vi "Actor Core.vi"(8 "error in":errorcluster, 11 "Electronic Load in":refnum<class "Electronic Load.lvclass">) -> (0 "error out":errorcluster, 3 "Actor out":refnum<class "Actor.lvclass">)   [LabVIEW 2019, in "Electronic Load.lvlib" / "Electronic Load.lvclass"]
doc: "The instrument actor core is only here to distribute panel resolution settings to children classes."
uses:
  Library/Electronic Load.lvclass
  C:/Users/Public/Documents/Development/builds/Instruments/Instruments.lvlibp/Library/Instruments.lvclass
  builds/Engine/Actor Framework.lvlibp/1abvi3w/vi.lib/ActorFramework/Actor/Actor.lvclass
  Custom Controls/E-Load Function.ctl
  Custom Controls/E-Load Mode.ctl
  Custom Controls/Trigger Settings.ctl
  Custom Controls/OCP Settings.ctl
  Custom Controls/Status_Flags.ctl
  Library/Electronic Load.lvclass/Electronic Load.ctl
  Electronic Load Messages/Write Output Enable Msg/Write Output Enable Msg.lvclass/Write Output Enable Msg.ctl
  Electronic Load Messages/Write Input Level Msg/Write Input Level Msg.lvclass/Write Input Level Msg.ctl
  Electronic Load Messages/Write Mode Msg/Write Mode Msg.lvclass/Write Mode Msg.ctl
  Electronic Load Messages/Write Slew Rate Msg/Write Slew Rate Msg.lvclass/Write Slew Rate Msg.ctl
  Electronic Load Messages/Write Pulse Enable Msg/Write Pulse Enable Msg.lvclass/Write Pulse Enable Msg.ctl
  Electronic Load Messages/Write Pulse Mode Msg/Write Pulse Mode Msg.lvclass/Write Pulse Mode Msg.ctl
  Electronic Load Messages/Write Pulse Initial Msg/Write Pulse Initial Msg.lvclass/Write Pulse Initial Msg.ctl
  Electronic Load Messages/Write Transient Msg/Write Transient Msg.lvclass/Write Transient Msg.ctl
  Electronic Load Messages/Write Pulse Sample Interval Msg/Write Pulse Sample Interval Msg.lvclass/Write Pulse Sample Interval Msg.ctl
  Electronic Load Messages/Write Pulse Width Msg/Write Pulse Width Msg.lvclass/Write Pulse Width Msg.ctl
  Electronic Load Messages/Write Pulse Delay Msg/Write Pulse Delay Msg.lvclass/Write Pulse Delay Msg.ctl
  Electronic Load Messages/Write Pulse Data Points Msg/Write Pulse Data Points Msg.lvclass/Write Pulse Data Points Msg.ctl
  Electronic Load Messages/Write Pulse Slew Msg/Write Pulse Slew Msg.lvclass/Write Pulse Slew Msg.ctl
  Electronic Load Messages/Write OCP Enable Msg/Write OCP Enable Msg.lvclass/Write OCP Enable Msg.ctl
  Electronic Load Messages/Write OCP Level Msg/Write OCP Level Msg.lvclass/Write OCP Level Msg.ctl
  Electronic Load Messages/Write OCP Delay Msg/Write OCP Delay Msg.lvclass/Write OCP Delay Msg.ctl
  Electronic Load Messages/Write Active Channel Msg/Write Active Channel Msg.lvclass/Write Active Channel Msg.ctl
  Private/GUI/Write Channels_Ref.vi
  Private/GUI/Write Settings_Ref.vi
  Private/GUI/Write Trigger_Ref.vi
  Private/GUI/Write Measured_Table.vi
  Private/GUI/Write OCP_Settings_Ref.vi
  Private/GUI/Write Trigger_TargetsRef.vi
  Private/GUI/Write Status_Flags_Ref.vi
  builds/Instruments/Instruments.lvlibp/Accessors/Write Snapshot Refnum.vi
  builds/Instruments/Instruments.lvlibp/Accessors/Write Graph_Ref.vi
  builds/Engine/Actor Framework.lvlibp/1abvi3w/vi.lib/ActorFramework/Message Enqueuer/Enqueue.vi
  Electronic Load Messages/Write Output Enable Msg/Write Output Enable Msg.lvclass
  Electronic Load Messages/Write Input Level Msg/Write Input Level Msg.lvclass
  Electronic Load Messages/Write Mode Msg/Write Mode Msg.lvclass
  Electronic Load Messages/Write Slew Rate Msg/Write Slew Rate Msg.lvclass
  Electronic Load Messages/Reset Eload Msg/Reset Eload Msg.lvclass
  Electronic Load Messages/Write Pulse Enable Msg/Write Pulse Enable Msg.lvclass
  Electronic Load Messages/Write Pulse Mode Msg/Write Pulse Mode Msg.lvclass
  Electronic Load Messages/Write Pulse Initial Msg/Write Pulse Initial Msg.lvclass
  Electronic Load Messages/Write Transient Msg/Write Transient Msg.lvclass
  Electronic Load Messages/Write Pulse Sample Interval Msg/Write Pulse Sample Interval Msg.lvclass
  Electronic Load Messages/Write Pulse Width Msg/Write Pulse Width Msg.lvclass
  Electronic Load Messages/Write Pulse Delay Msg/Write Pulse Delay Msg.lvclass
  Electronic Load Messages/Write Pulse Data Points Msg/Write Pulse Data Points Msg.lvclass
  Electronic Load Messages/Write Pulse Slew Msg/Write Pulse Slew Msg.lvclass
  Electronic Load Messages/Write OCP Enable Msg/Write OCP Enable Msg.lvclass
  Electronic Load Messages/Write OCP Level Msg/Write OCP Level Msg.lvclass
  Electronic Load Messages/Write OCP Delay Msg/Write OCP Delay Msg.lvclass
  Electronic Load Messages/Write Active Channel Msg/Write Active Channel Msg.lvclass
  builds/Instruments/Instruments.lvlibp/Library/Instruments.lvclass
  builds/Instruments/Instruments.lvlibp/Instruments Messages/Take Snapshot Msg/Take Snapshot Msg.lvclass
panel:
  out "Status":T1
  in  "Reset":bool
  in  "Pulse":bool
  in  "Active Device":u16(ring)
  out "Control":enum32{"Constant", "Pulsed"}(tab)
  in  "Settings":T2
  in  "OCP Settings":T4
  in  "Active Channel":u16(ring)
  in  "Trigger Settings":T5 {"Delay" format="%#_g s"; "Interval" format="%#_g s"; "Width" format="%#_g s"}
  in  "Trigger Targets":i32(listbox)=-1
  in  "View":enum16{"Continuous", "Snapshot", "Table"}(ring)
  in  "Operation":enum16{"Constant", "Pulsed"}(ring)
  out "Display Format":enum32{"Continuous", "Snapshot", "Table"}(tab)
  out "Continuous Plot":waveform(dbl)[](graph)
  out "Snapshot Plot":waveform(dbl)[](graph)
  out "Measured Table":i32(listbox)
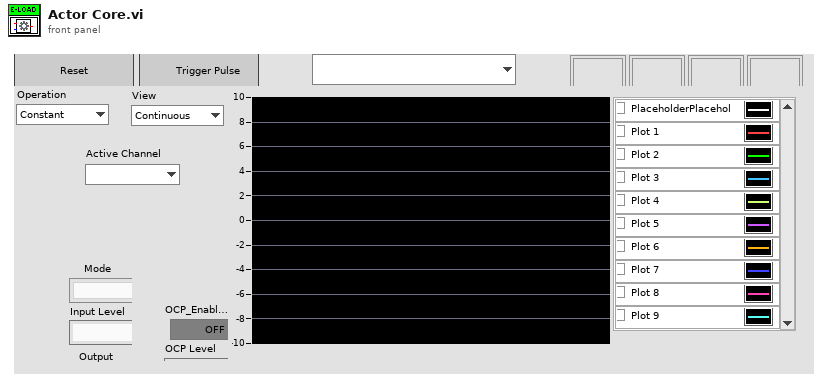
[diagram p1: front panel]
types:
  T1 = typedef "Electronic Load.lvlib/Electronic Load.lvclass/Status_Flags.ctl" = cluster{"Interlock":bool, "OVP":bool, "OCP":bool, "Output":bool}
  T2 = typedef "Electronic Load.lvlib/Electronic Load.lvclass/E-Load Function.ctl" = cluster{"Mode":T3, "Input Level":dbl, "Output":bool, "Slew Rate":dbl}
  T3 = typedef "Electronic Load.lvlib/Electronic Load.lvclass/E-Load Mode.ctl" = enum16{"Current", "Resistance", "Voltage"}
  T4 = typedef "Electronic Load.lvlib/Electronic Load.lvclass/OCP Settings.ctl" = cluster{"OCP_Enabled":bool, "OCP Level":dbl, "OCP Delay":dbl}
  T5 = typedef "Electronic Load.lvlib/Electronic Load.lvclass/Trigger Settings.ctl" = cluster{"Mode":T3, "Initial":dbl, "Transient":dbl, "Interval":dbl, "Width":dbl, "Delay":dbl, "Data Pts":i32, "Slew Rate":dbl}
  T6 = cluster{"Pnl Actor":refnum<event-registration>, "Event Registration Refnum":refnum<event-registration>}
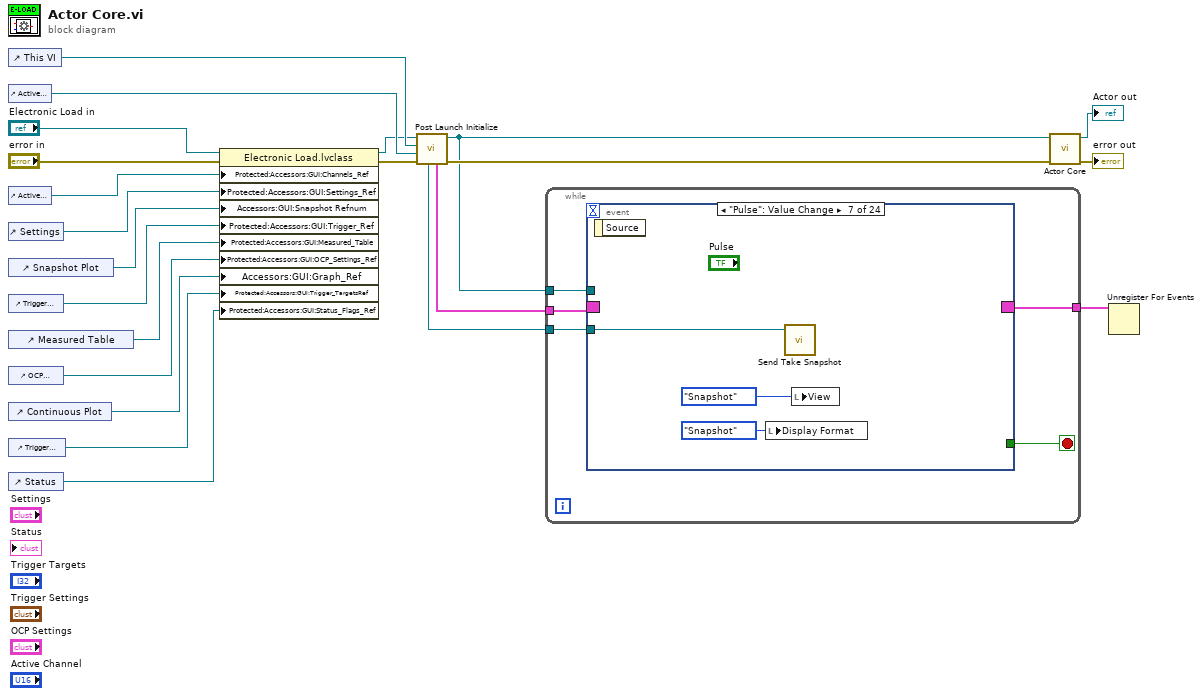
[diagram p0: block diagram]
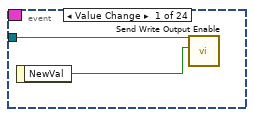
[diagram p2: hidden frame]
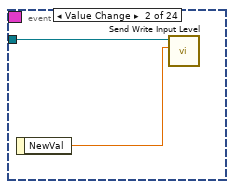
[diagram p3: hidden frame]
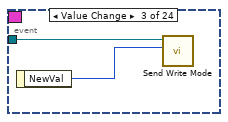
[diagram p4: hidden frame]
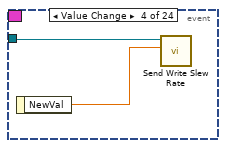
[diagram p5: hidden frame]
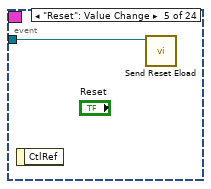
[diagram p6: hidden frame]
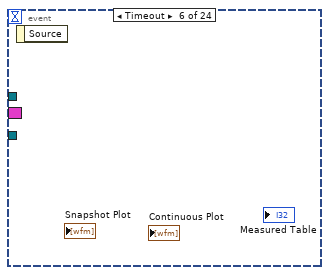
[diagram p7: hidden frame]
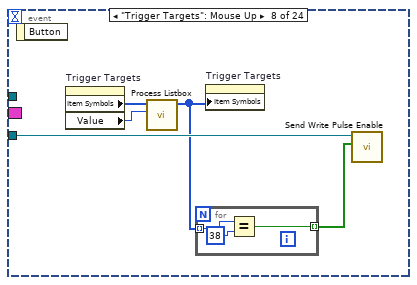
[diagram p8: hidden frame]
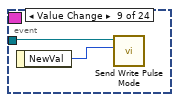
[diagram p9: hidden frame]
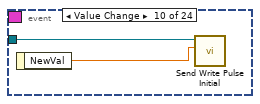
[diagram p10: hidden frame]
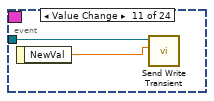
[diagram p11: hidden frame]
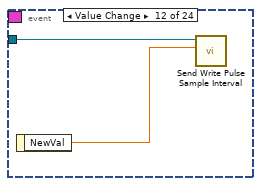
[diagram p12: hidden frame]
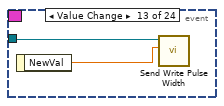
[diagram p13: hidden frame]
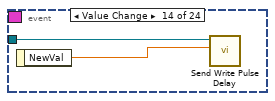
[diagram p14: hidden frame]
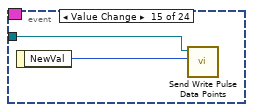
[diagram p15: hidden frame]
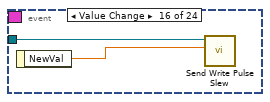
[diagram p16: hidden frame]
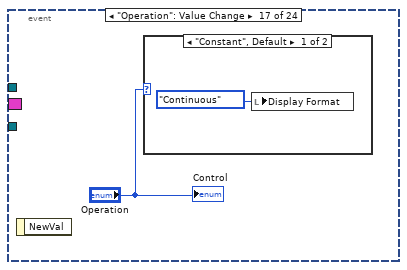
[diagram p17: hidden frame]
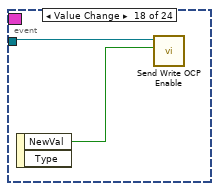
[diagram p19: hidden frame]
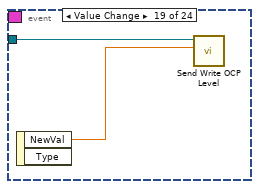
[diagram p20: hidden frame]
diagram:
  n1 = control-ref of="This VI"() -> (w19:refnum<vi>)
  n2 = control-ref of="Active Device"() -> (w20:refnum<vi>)
  n3 = control-ref of="Active Channel"() -> (w10:refnum<vi>)
  n4 = control-ref of="Settings"() -> (w9:refnum<vi>)
  n5 = control-ref of="Snapshot Plot"() -> (w8:refnum<vi>)
  n6 = control-ref of="Trigger Settings"() -> (w7:refnum<vi>)
  n7 = control-ref of="Measured Table"() -> (w5:refnum<vi>)
  n8 = control-ref of="OCP Settings"() -> (w4:refnum<vi>)
  n9 = control-ref of="Continuous Plot"() -> (w3:refnum<vi>)
  n10 = control-ref of="Trigger Targets"() -> (w2:refnum<vi>)
  n11 = control-ref of="Status"() -> (w1:refnum<vi>)
  n12 = property class="Electronic Load.lvclass"(reference="Electronic Load in", error in="error in", "Protected:Accessors:GUI:Channels_Ref"=w10, "Protected:Accessors:GUI:Settings_Ref"=w9, "Accessors:GUI:Snapshot Refnum"=w8, "Protected:Accessors:GUI:Trigger_Ref"=w7, "Protected:Accessors:GUI:Measured_Table"=w5, "Protected:Accessors:GUI:OCP_Settings_Ref"=w4, "Accessors:GUI:Graph_Ref"=w3, "Protected:Accessors:GUI:Trigger_TargetsRef"=w2, "Protected:Accessors:GUI:Status_Flags_Ref"=w1) -> (reference out=w15:refnum<class "Electronic Load.lvclass">, error out=w16:errorcluster)
  n13 = call "Post Launch Initialize.vi"("error in"=w16, "Active Device"=w20, "GUI Reference"=w19, "Instruments in"=w15) -> ("error out"=w14:errorcluster, "Instruments out"=w6:refnum<class "Electronic Load.lvclass">, "Registered Events"=w13:T6, "Self Enqueuer"=w12:refnum<class "Message Enqueuer.lvclass">)  [unwired: 4 in]
  n14 = while {
    tunnel: w13 -> [w27]
    tunnel: w12 -> [w23]
    tunnel: w6 -> [w24]
    tunnel: [w26] -> w11
    stop <- w25 stop-if-true
    n15 = event shown="[6] \"Pulse\": Value Change" {
      selector: w27 -> [_ _ _ _ _ _ _ _ _ _ _ _ _ _ _ _ _ _ _ _ _ _ _ _]
      dyn-events: [_ _ _ _ _ _ _ _ _ _ _ _ _ _ _ _ _ _ _ _ _ _ _ _] -> w26
      timeout: _ -> [_ _ _ _ _ _ _ _ _ _ _ _ _ _ _ _ _ _ _ _ _ _ _ _]
      tunnel: [_ _ _ _ _ _ _ _ _ _ _ _ _ _ _ _ _ _ _ _ TRUE _ _ _] -> w25
      tunnel: w24 -> [_ _ _ _ _ _ _ _ _ _ _ _ _ _ _ _ _ _ _ _ _ _ _ w78]
      tunnel: w23 -> [w29 w31 w33 w35 w36 _ w39 w44 w49 w51 w53 w55 w57 w59 w61 w63 _ w67 w69 w71 _ w74 _ _]
      event Value Change {
        n16 = event-data() -> ("NewVal"=w28:bool)  [unwired: 1 in]
        n17 = call "Send Write Output Enable.vi"("Output"=w28, "Message Enqueuer"=w29) -> ()  [unwired: 8 in, 2 out]
      }
      event Value Change {
        n18 = event-data() -> ("NewVal"=w30:dbl)  [unwired: 1 in]
        n19 = call "Send Write Input Level.vi"("Input Level"=w30, "Message Enqueuer"=w31) -> ()  [unwired: 8 in, 2 out]
      }
      event Value Change {
        n20 = event-data() -> ("NewVal"=w32:T3)  [unwired: 1 in]
        n21 = call "Send Write Mode.vi"("Mode"=w32, "Message Enqueuer"=w33) -> ()  [unwired: 8 in, 2 out]
      }
      event Value Change {
        n22 = event-data() -> ("NewVal"=w34:dbl)  [unwired: 1 in]
        n23 = call "Send Write Slew Rate.vi"("Slew Rate"=w34, "Message Enqueuer"=w35) -> ()  [unwired: 8 in, 2 out]
      }
      event "Reset": Value Change {
        n24 = event-data() -> ()  [unwired: 1 in, 1 out]
        n25 = call "Send Reset Eload.vi"("Message Enqueuer"=w36) -> ()  [unwired: 9 in, 2 out]
      }
      event Timeout {
        n26 = event-data() -> ()  [unwired: 1 in, 1 out]
      }
      event "Pulse": Value Change {
        n27 = event-data() -> ()  [unwired: 1 in, 1 out]
        n28 = local write "Display Format"(enum32{"Continuous", "Snapshot", "Table"}."Snapshot" ("Display Format")) -> ()
        n29 = call "Send Take Snapshot.vi"("Message Enqueuer"=w39) -> ()  [unwired: 9 in, 2 out]
        n30 = local write "View"(enum16{"Continuous", "Snapshot", "Table"}."Snapshot" ("View")) -> ()
      }
      event "Trigger Targets": Mouse Up {
        n31 = event-data() -> ()  [unwired: 1 in, 1 out]
        n32 = property on="Trigger Targets" class="LstBox (strict)"() -> ("Item Symbols"=w42:i32[], "Value"=w40:i32)  [unwired: 2 in, 2 out]
        n33 = call "Process Listbox.vi"("Select"=w40, "Item Symbols in"=w42) -> ("Item Symbols out"=w41:i32[])  [unwired: 9 in]
        n34 = for {
          tunnel: w41 -> [w47] mode=indexing
          tunnel: [w45] -> w43 mode=indexing
          n35 = Equal?(x=w47, y=38) -> (x = y?=w45:bool)
        }
        n36 = property on="Trigger Targets" class="LstBox (strict)"("Item Symbols"=w41) -> ()  [unwired: 2 in, 2 out]
        n37 = call "Send Write Pulse Enable.vi"("Chan_Trig_En"=w43, "Message Enqueuer"=w44) -> ()  [unwired: 8 in, 2 out]
      }
      event Value Change {
        n38 = event-data() -> ("NewVal"=w48:T3)  [unwired: 1 in]
        n39 = call "Send Write Pulse Mode.vi"("Pulse Mode"=w48, "Message Enqueuer"=w49) -> ()  [unwired: 8 in, 2 out]
      }
      event Value Change {
        n40 = event-data() -> ("NewVal"=w50:dbl)  [unwired: 1 in]
        n41 = call "Send Write Pulse Initial.vi"("Pulse Initial"=w50, "Message Enqueuer"=w51) -> ()  [unwired: 8 in, 2 out]
      }
      event Value Change {
        n42 = event-data() -> ("NewVal"=w52:dbl)  [unwired: 1 in]
        n43 = call "Send Write Transient.vi"("Transient"=w52, "Message Enqueuer"=w53) -> ()  [unwired: 8 in, 2 out]
      }
      event Value Change {
        n44 = event-data() -> ("NewVal"=w54:dbl)  [unwired: 1 in]
        n45 = call "Send Write Pulse Sample Interval.vi"("Sample Interval"=w54, "Message Enqueuer"=w55) -> ()  [unwired: 8 in, 2 out]
      }
      event Value Change {
        n46 = event-data() -> ("NewVal"=w56:dbl)  [unwired: 1 in]
        n47 = call "Send Write Pulse Width.vi"("Pulse Width"=w56, "Message Enqueuer"=w57) -> ()  [unwired: 8 in, 2 out]
      }
      event Value Change {
        n48 = event-data() -> ("NewVal"=w58:dbl)  [unwired: 1 in]
        n49 = call "Send Write Pulse Delay.vi"("Delay"=w58, "Message Enqueuer"=w59) -> ()  [unwired: 8 in, 2 out]
      }
      event Value Change {
        n50 = event-data() -> ("NewVal"=w60:i32)  [unwired: 1 in]
        n51 = call "Send Write Pulse Data Points.vi"("Data Pts"=w60, "Message Enqueuer"=w61) -> ()  [unwired: 8 in, 2 out]
      }
      event Value Change {
        n52 = event-data() -> ("NewVal"=w62:dbl)  [unwired: 1 in]
        n53 = call "Send Write Pulse Slew.vi"("Slew"=w62, "Message Enqueuer"=w63) -> ()  [unwired: 8 in, 2 out]
      }
      event "Operation": Value Change {
        n54 = event-data() -> ()  [unwired: 1 in, 1 out]
        n55 = case shown="\"Constant\", Default" "Operation" {
          frame "Constant", Default {
            n56 = local write "Display Format"(enum32{"Continuous", "Snapshot", "Table"}."Continuous" ("Display Format")) -> ()
          }
          frame "Pulsed" {
          }
        }
        "Control" <- "Operation"
      }
      event Value Change {
        n57 = event-data() -> ("NewVal"=w66:bool)  [unwired: 1 in, 1 out]
        n58 = call "Send Write OCP Enable.vi"("OCP Enable"=w66, "Message Enqueuer"=w67) -> ()  [unwired: 8 in, 2 out]
      }
      event Value Change {
        n59 = event-data() -> ("NewVal"=w68:dbl)  [unwired: 1 in, 1 out]
        n60 = call "Send Write OCP Level.vi"("OCP Level"=w68, "Message Enqueuer"=w69) -> ()  [unwired: 8 in, 2 out]
      }
      event Value Change {
        n61 = event-data() -> ("NewVal"=w70:dbl)  [unwired: 1 in]
        n62 = call "Send Write OCP Delay.vi"("Delay"=w70, "Message Enqueuer"=w71) -> ()  [unwired: 8 in, 2 out]
      }
      event User Event {
        n63 = event-data() -> ()  [unwired: 1 in, 1 out]
      }
      event "Active Channel": Value Change {
        n64 = event-data() -> ("NewVal"=w73:u16)  [unwired: 1 in]
        n65 = call "Send Write Active Channel.vi"("Active Channel"=w73, "Message Enqueuer"=w74) -> ()  [unwired: 8 in, 2 out]
      }
      event "View": Value Change {
        n66 = event-data() -> ()  [unwired: 1 in, 1 out]
        "Display Format" <- "View"
      }
      event "Active Device": Value Change {
        n67 = event-data() -> ("OldVal"=w77:u16, "NewVal"=w76:u16)  [unwired: 1 in]
        n68 = call "Trigger Instr View.vi"("New Value"=w76, "Old Value"=w77, "Instruments in"=w78) -> ()  [unwired: 7 in, 2 out]
      }
    }
  }
  n69 = call-parent "Actor Core.vi"("error in"=w14, "Instruments in"=w6) -> ("error out"=→"error out":errorcluster, "Actor out"=→"Actor out":refnum<class "Actor.lvclass">)  [unwired: 8 in]
  n70 = Unregister For Events(event registration refnum=w11) -> ()  [unwired: 1 in, 1 out]
